vi "CloseClk.vi"(8 "error in (no error)":errorcluster, 10 "ClkName":string, 11 "Local in":refnum<class "Local.lvclass">) -> (0 "error out":errorcluster, 3 "Local out":refnum<class "Local.lvclass">)   [LabVIEW 2014, in "SyncPlugins.lvlib" / "Local.lvclass"]
uses:
  Local.lvclass
  SyncPluginBase/SyncPluginBase.lvclass
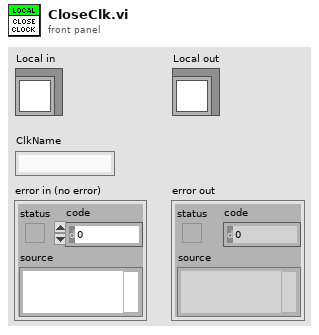
[diagram p1: front panel]
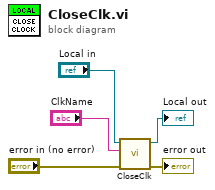
[diagram p0: block diagram]
diagram:
  n1 = call-parent "CloseClk.vi"("error in (no error)"="error in (no error)", "ClkName"="ClkName", "SyncPluginBase in"="Local in") -> ("error out"=→"error out":errorcluster, "SyncPluginBase out"=→"Local out":refnum<class "Local.lvclass">)  [unwired: 7 in]
